vi "check_mouse_input.vi"(1 "input cluster":T1) -> (0 "output cluster":T2)   [LabVIEW 2010]
uses:
  <vilib>/Utility/inputDevices.llb/mouseAcquire.vi
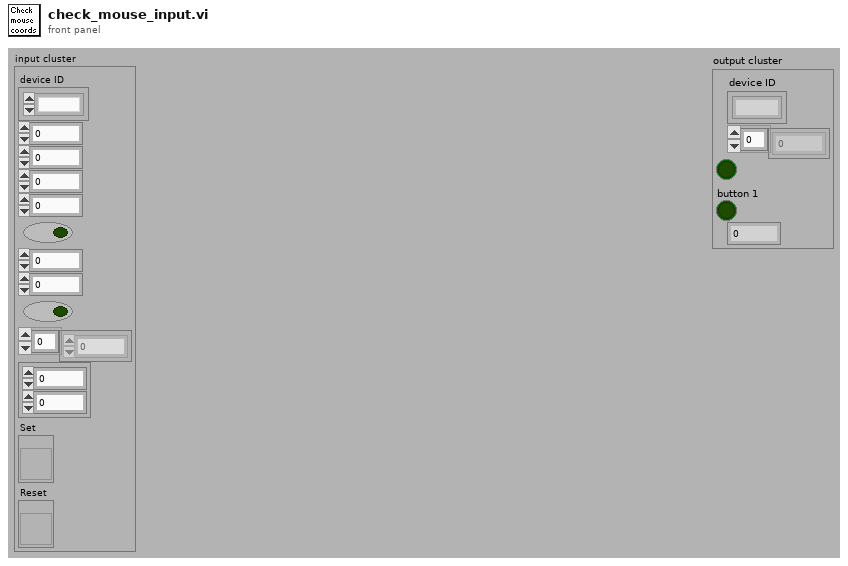
[diagram p1: front panel]
types:
  T1 = cluster{"device ID":refnum<k1>, i32, i32, u32, u32, bool, i32, i32, bool, dbl[], cluster{i32, i32}, "Set":refnum<vi>, "Reset":refnum<vi>}
  T2 = cluster{"device ID":refnum<k1>, dbl[], bool, "button 1":bool, i32}
  T3 = cluster{"Horizontal":i32, "Vertical":i32, "Scrolling":i32}
  T4 = cluster{"button 1":bool, "button 2":bool, "button 3":bool, "button 4":bool}
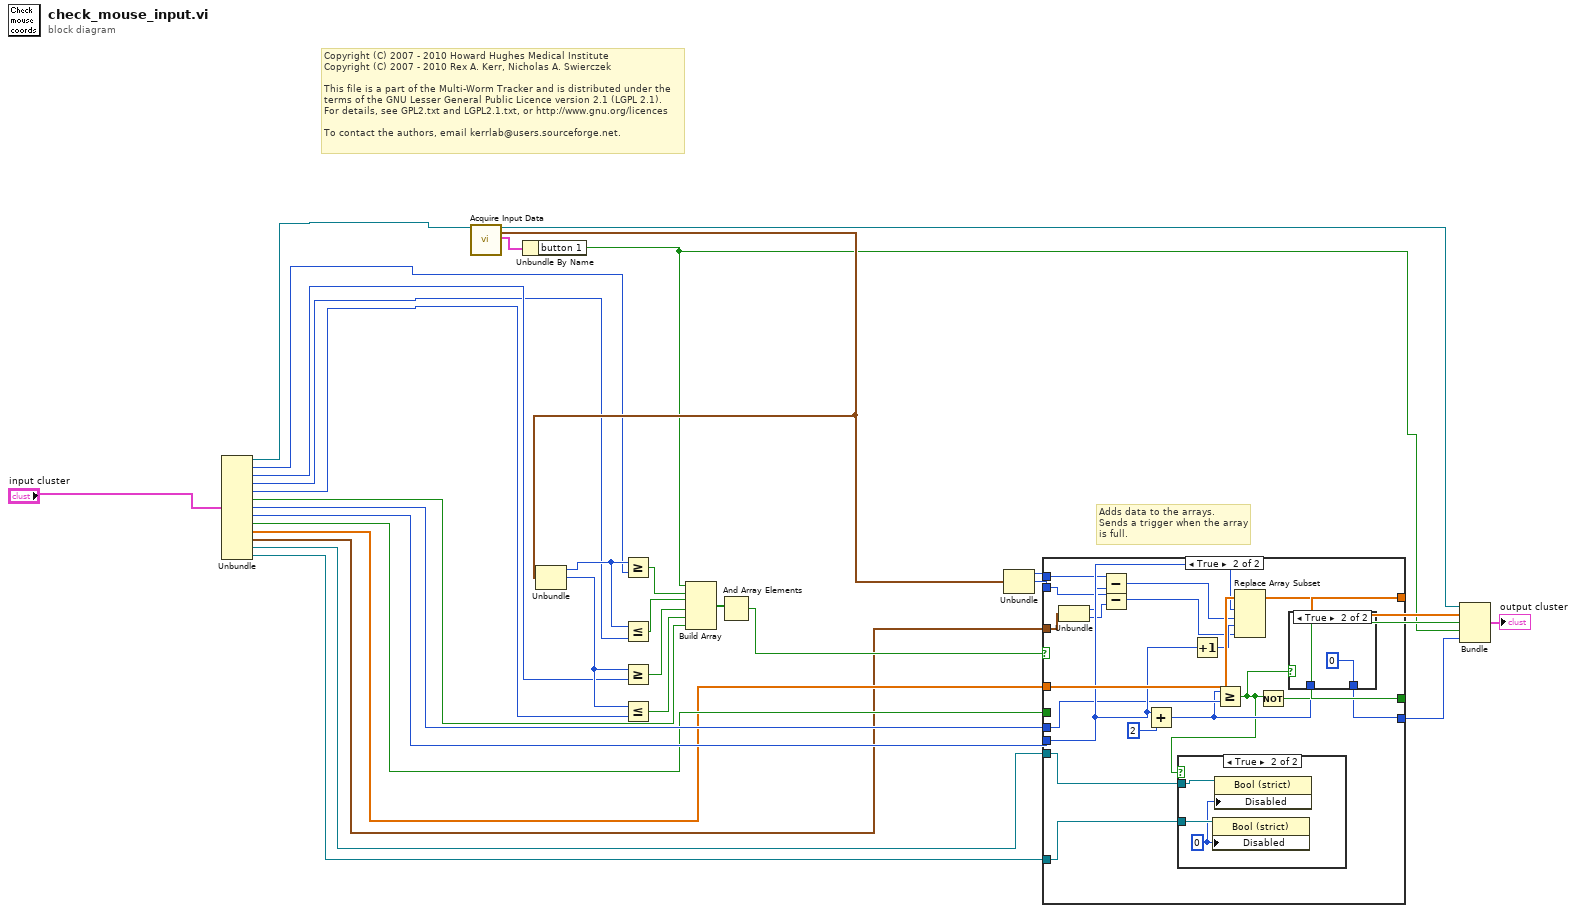
[diagram p0: block diagram]
diagram:
  # "Copyright (C) 2007 - 2010 Howard Hughes Medical Institute\nCopyright (C) 2007 - 2010 Rex A. Kerr, Nicholas A. Swierczek\n \nThis file is a part of the Multi-Worm Tracker and is distributed under the\nterms of the GNU Lesser General Public Licence version 2.1 (LGPL 2.1).\nFor details, see GPL2.txt and LGPL2.1.txt, or http://www.gnu.org/licences\n \nTo contact the authors, email kerrlab@users.sourceforge.net."
  # "Adds data to the arrays.\nSends a trigger when the array\nis full."
  n1 = Unbundle("input cluster") -> ("device ID"=w21:refnum<k1>, w20:i32, w19:i32, w18:u32, w17:u32, w16:bool, w15:i32, w14:i32, w13:bool, w12:dbl[], w9:cluster{i32, i32}, "Set"=w6:refnum<vi>, "Reset"=w1:refnum<vi>)
  n2 = call-poly <vilib>:"Acquire Input Data.vi"("device ID"=w21) -> ("device ID"=w7:refnum<k1>, "axis info"=w26:T3, "button info"=w8:T4)  [unwired: 15 in, 1 out]
  n3 = Unbundle By Name(w8) -> ("button 1"=w4:bool)
  n4 = Unbundle(w26) -> ("Horizontal"=w25:i32, "Vertical"=w24:i32)  [unwired: 1 out]
  n5 = Greater Or Equal?(x=w25, y=w20) -> (x >= y?=w32:bool)
  n6 = Less Or Equal?(x=w25, y=w18) -> (x <= y?=w31:bool)
  n7 = Greater Or Equal?(x=w24, y=w19) -> (x >= y?=w30:bool)
  n8 = Less Or Equal?(x=w24, y=w17) -> (x <= y?=w29:bool)
  n9 = Build Array(w4, w32, w31, w30, w29, w16) -> (w28:bool[])
  n10 = And Array Elements(Boolean array=w28) -> (logical AND=w27:bool)
  n11 = Unbundle(w26) -> ("Horizontal"=w23:i32, "Vertical"=w22:i32)  [unwired: 1 out]
  n12 = case shown="True" w27 {
    tunnel: w23 -> [_ w42]
    tunnel: w22 -> [_ w41]
    tunnel: w14 -> [w35 w51]
    tunnel: [w35 w39] -> w5
    tunnel: w12 -> [w34 w54]
    tunnel: [w34 w52] -> w10
    tunnel: w15 -> [_ w49]
    tunnel: [w33 w48] -> w11
    tunnel: w13 -> [w33 _]
    tunnel: w9 -> [_ w47]
    tunnel: w6 -> [_ w36]
    tunnel: w1 -> [_ w37]
    frame False {
    }
    frame True {
      n13 = Unbundle(w47) -> (w44:i32, w43:i32)
      n14 = Subtract(x=w42, y=w44) -> (x-y=w46:i32)
      n15 = Subtract(x=w41, y=w43) -> (x-y=w45:i32)
      n16 = Add(x=w51, y=2) -> (x+y=w40:i32)
      n17 = Increment(x=w51) -> (x+1=w53:i32)
      n18 = Greater Or Equal?(x=w40, y=w49) -> (x >= y?=w38:bool)
      n19 = case shown="True" w38 {
        tunnel: w37 -> [_ w57]
        tunnel: w36 -> [_ w56]
        frame False {
        }
        frame True {
          w55 = u8 0 ("Disabled")
          n20 = property class="Bool (strict)"(reference=w57, "Disabled"=w55) -> ()  [unwired: 1 in, 2 out]
          n21 = property class="Bool (strict)"(reference=w56, "Disabled"=w55) -> ()  [unwired: 1 in, 2 out]
        }
      }
      n22 = Replace Array Subset(array=w54, new element #1=w46, index #1=w51, new element #2=w45, index #2=w53) -> (w52:dbl[])
      n23 = Not(x=w38) -> (.not. x?=w48:bool)
      n24 = case shown="True" w38 {
        tunnel: w40 -> [w58 _]
        tunnel: [w58 0] -> w39
        frame False {
        }
        frame True {
        }
      }
    }
  }
  n25 = Bundle("device ID"=w7, w10, w11, "button 1"=w4, w5) -> (→"output cluster":T2)  [unwired: 1 in]
